vi "Sample Transfer Override Vacuum State.vi"(8 "error in (no error)":errorcluster, 10 "State (Plateau)":T1=enum."Plateau", 11 "cRIO-CO2 in":refnum<class "cRIO-CO2.lvclass">) -> (0 "error out":errorcluster, 3 "cRIO-CO2 out":refnum<class "cRIO-CO2.lvclass">)   [LabVIEW 2015, in "cRIO-Carbondioxide.lvlib" / "cRIO-CO2.lvlib" / "cRIO-CO2.lvclass"]
uses:
  cRIO-CO2.lvclass
  Controls/Vacuum State Enumerator.ctl
  <vilib>/ActorFramework/Message Enqueuer/Message Priority.ctl
  cRIO-CO2.lvclass/cRIO-CO2.ctl
  cRIO Vacuum Messages/Override State Msg/Override State Msg.lvclass/Override State Msg.ctl
  <vilib>/ActorFramework/Message Enqueuer/Message Enqueuer.lvclass/Message Enqueuer.ctl
  <vilib>/ActorFramework/Message Enqueuer/Enqueue.vi
  <vilib>/ActorFramework/Message Priority Queue/Priority Enqueue.vi
  cRIO Vacuum Messages/Override State Msg/Override State Msg.lvclass
  <vilib>/ActorFramework/Message Enqueuer/Message Enqueuer.lvclass
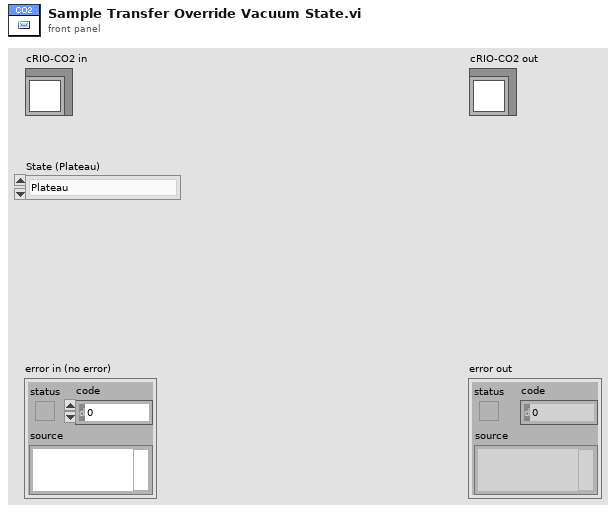
[diagram p1: front panel]
types:
  T1 = typedef "Vacuum State Enumerator.ctl" = enum16{"Pressure Rising", "Plateau", "Pressure Dropping", "Valley", "Low Valley", "Leak", "Unknown"}
  T2 = typedef "Actor Framework.lvlib/Message Enqueuer.lvclass/Message Priority.ctl" = enum16{"Low", "Normal", "High"}
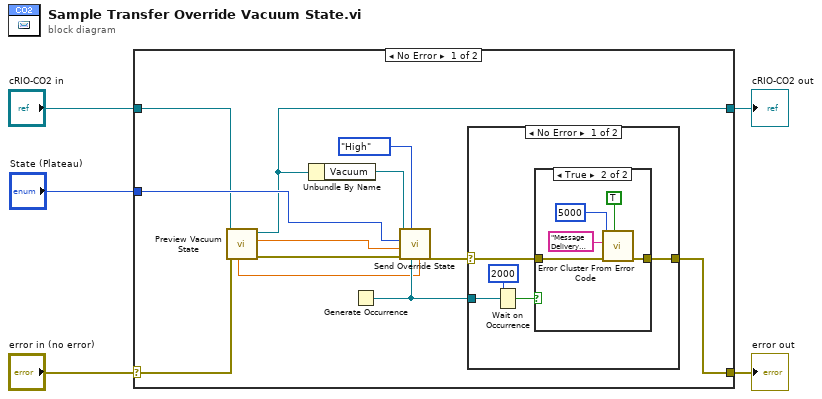
[diagram p0: block diagram]
diagram:
  n1 = case shown="No Error" "error in (no error)" {
    selector: "error in (no error)" -> [w13 w31]
    tunnel: [w7 w31] -> w4
    tunnel: [w11 w30] -> w2
    tunnel: "cRIO-CO2 in" -> [w12 w30]
    tunnel: "State (Plateau)" -> [w14 _]
    frame No Error {
      n2 = call "Preview Vacuum State.vi"("error in (no error)"=w13, "cRIO-CO2 in"=w12) -> ("error out"=w17:errorcluster, "Pressure (mBar)"=w15:dbl, "cRIO-CO2 out"=w11:refnum<class "cRIO-CO2.lvclass">, "Raw Pressure"=w6:dbl)  [unwired: 3 in, 3 out]
      n3 = Unbundle By Name(w11) -> ("Vacuum"=w16:refnum<class "Message Enqueuer.lvclass">)
      n4 = Generate Occurrence() -> (w9:refnum<k4>)
      n5 = call "Send Override State.vi"("Raw Pressure"=w6, "occurrence"=w9, "Message Priority (Normal)"=Message_Priority."High", "error in (no error)"=w17, "Pressure"=w15, "State"=w14, "Message Enqueuer"=w16) -> ("error out"=w8:errorcluster)  [unwired: 3 in, 1 out]
      n6 = case shown="No Error" w8 {
        selector: w8 -> [w19 w29]
        tunnel: w9 -> [w21 _]
        tunnel: [w18 w29] -> w7
        frame No Error {
          n7 = Wait on Occurrence(2:w21, 3:2000 ("ms timeout (-1)")) -> (0:w20:bool)  [unwired: 1 in]
          n8 = case shown="True" w20 {
            tunnel: w19 -> [w23 w28]
            tunnel: [w23 w27] -> w18
            frame False {
            }
            frame True {
              n9 = call <vilib>:"Error Cluster From Error Code.vi"("show call chain? (False)"=TRUE, "error in (no error)"=w28, "error message (\"\")"="Message Delivery Occurrence timed out" ("error message (\"\")"), "error code (0)"=5000) -> ("error out"=w27:errorcluster)  [unwired: 5 in]
            }
          }
        }
        frame Error {
        }
      }
    }
    frame Error {
    }
  }
  "error out" <- w4
  "cRIO-CO2 out" <- w2
